vi "XSuperLink Demo.vi"() -> ()   [LabVIEW 2011]
uses:
  xcontrol/XSuperLink.xctl
panel:
  in  "Stop":bool
  out "E-mail":string(xcontrol) caption="E-mail-->"
  out "http":string(xcontrol) caption="http-->"
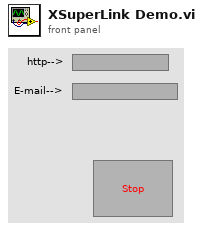
[diagram p1: front panel]
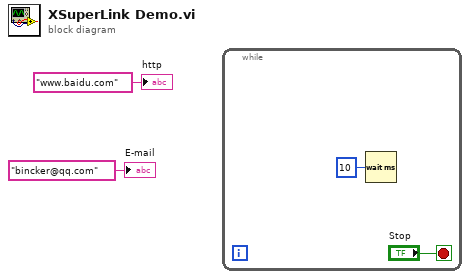
[diagram p0: block diagram]
diagram:
  n1 = while {
    stop <- "Stop" stop-if-true
    n2 = Wait (ms)(milliseconds to wait=u32 10 ("等待时间（毫秒）")) -> ()  [unwired: 1 out]
  }
  "http" <- "www.baidu.com" ("http")
  "E-mail" <- "bincker@qq.com" ("E-mail")
